vi "Check Higher Fault.vi"(8 "error in (no error)":errorcluster, 10 "Input Values":sgl[](array[numeric]), 11 "AILimitConfig":T1(array[cluster])) -> (0 "error out":errorcluster, 2 "HF Events":string[](array[string]), 3 "HF Channel":string[](array[string]))   [LabVIEW 2018]
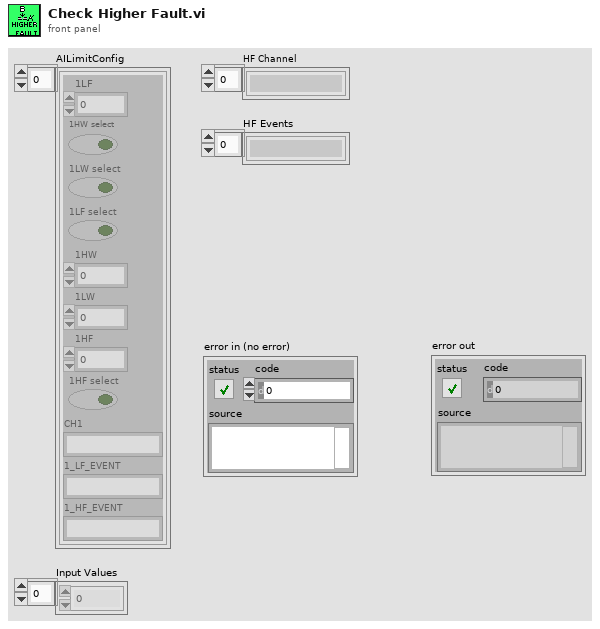
[diagram p1: front panel]
types:
  T1 = cluster{"1LF":dbl, "1HW select":bool, "1LW select":bool, "1LF select":bool, "1HW":dbl, "1LW":dbl, "1HF":dbl, "1HF select":bool, "CH1":string, "1_LF_EVENT":string, "1_HF_EVENT":string}[]
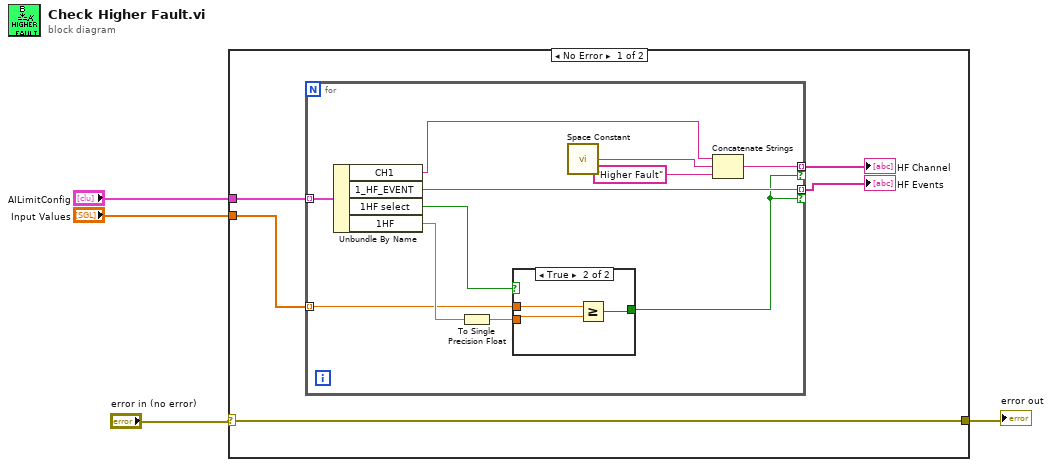
[diagram p0: block diagram]
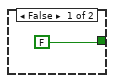
[diagram p2: hidden frame]
diagram:
  n1 = case shown="No Error" "error in (no error)" {
    selector: "error in (no error)" -> [w5 w25]
    tunnel: "Input Values" -> [w9 _]
    tunnel: "AILimitConfig" -> [w6 _]
    tunnel: [w5 w25] -> w1
    frame No Error {
      n2 = for {
        tunnel: w6 -> [w20] mode=indexing
        tunnel: [w19] -> w8 mode=indexing if=w11
        tunnel: w9 -> [w16] mode=indexing
        tunnel: [w12] -> w7 mode=indexing if=w11
        n3 = Unbundle By Name(w20) -> ("CH1"=w13:string, "1_HF_EVENT"=w19:string, "1HF select"=w18:bool, "1HF"=w17:dbl)
        n4 = To Single Precision Float(number=w17) -> (single precision float=w10:sgl)
        n5 = case shown="True" w18 {
          tunnel: w16 -> [_ w24]
          tunnel: w10 -> [_ w23]
          tunnel: [FALSE w22] -> w11
          frame False {
          }
          frame True {
            n6 = Greater Or Equal?(x=w24, y=w23) -> (x >= y?=w22:bool)
          }
        }
        n7 = call <vilib>:"Space Constant.vi"() -> ("String"=w15:string)
        n8 = Concatenate Strings(w13, w15, "Higher Fault" ("string")) -> (w12:string)
      }
      "HF Events" <- w8
      "HF Channel" <- w7
    }
    frame Error {
    }
  }
  "error out" <- w1
